vi "bson_find.vi"(9 "name":string, 10 "obj in":T1, 11 "bson_iterator":i32) -> (2 "obj out":T1, 3 "bson_iterator out":i32)   [LabVIEW 2013]
uses:
  bson.ctl
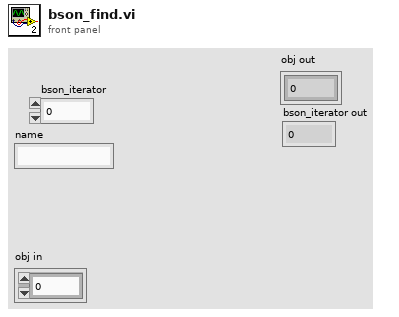
[diagram p1: front panel]
types:
  T1 = typedef "bson.ctl" = cluster{i32}
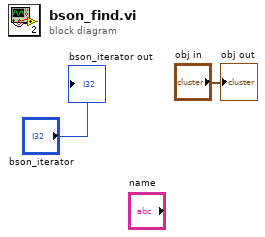
[diagram p0: block diagram]
diagram:
  "obj out" <- "obj in"
  "bson_iterator out" <- "bson_iterator"
